vi "Property Write.vi"(4 "error in (no error)":errorcluster, 5 "Value":bool, 6 "Container State":T3, 7 "Display State In":T1) -> (0 "error out":errorcluster, 3 "Display State Out":T1)   [LabVIEW 2015, in "KPropertyTable.xctl"]
uses:
  KPropertyTable.xctl
  <vilib>/_xctls/Container State.ctl
  State.vi
  DataType.ctl
  <vilib>/_xctls/XControlSupport.lvlib
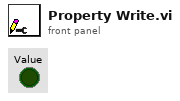
[diagram p1: front panel]
types:
  T1 = typedef "KPropertyTable.xctl/State.vi" = cluster{"show categories":bool, "table":refnum<vi>, "items":i32[], "enum row":i32, "edit type":T2, "edit row":i32, "max rows":i32, "scrollbar":bool}
  T2 = typedef "KPropertyTable.xctl/DataType.ctl" = enum16{"String", "Enum", "Int", "Double", "Boolean", "Ring", "Formula"}
  T3 = typedef "XControlSupport.lvlib/Container State.ctl" = cluster{"Indicator?":bool, "Run Mode?":bool, " Refnum":refnum<vi>}
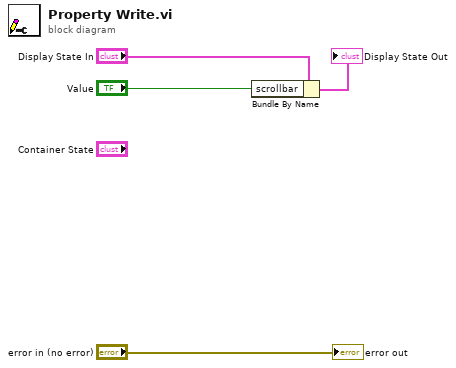
[diagram p0: block diagram]
diagram:
  n1 = Bundle By Name(cluster="Display State In", "scrollbar"="Value") -> (→"Display State Out":T1)
  "error out" <- "error in (no error)"
